vi "Show GUI if Debug.vi"(8 "error in (no error)":errorcluster, 11 "Module in":refnum<class "Module.lvclass">) -> (0 "error out":errorcluster, 3 "Module out":refnum<class "Module.lvclass">)   [LabVIEW 2020, in "Volatus.lvlib" / "Module.lvclass"]
uses:
  Module.lvclass
  Module.lvclass/Module.ctl
  MessageQ/MessageQ.lvclass/MessageQ.ctl
  Self Q.vi
  MessageQ/Send.vi
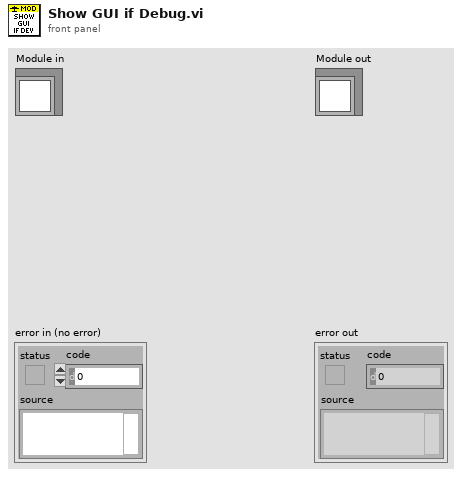
[diagram p1: front panel]
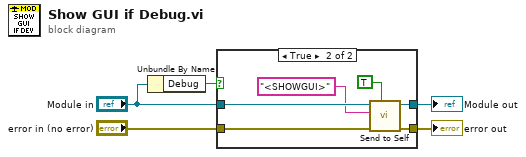
[diagram p0: block diagram]
diagram:
  n1 = Unbundle By Name("Module in") -> ("Debug"=w1:bool)
  n2 = case shown="True" w1 {
    tunnel: "Module in" -> [w7 w11]
    tunnel: "error in (no error)" -> [w6 w10]
    tunnel: [w7 w13] -> w4
    tunnel: [w6 w12] -> w3
    frame False {
    }
    frame True {
      n3 = call "Send to Self.vi"("High Priority (F)"=TRUE, "error in (no error)"=w10, "Message ID"="<SHOWGUI>", "Module in"=w11) -> ("error out"=w12:errorcluster, "Module out"=w13:refnum<class "Module.lvclass">)  [unwired: 6 in]
    }
  }
  "error out" <- w3
  "Module out" <- w4
